vi "subFD_FLP Filtering.vi"() -> ()   [LabVIEW 2023]
uses:
  <vilib>/addons/Digital Filter Design/_Objects.llb/DFD Filter Obj.ctl
  <vilib>/addons/Digital Filter Design/_Objects.llb/DFD Filter Coef.ctl
  <vilib>/addons/Digital Filter Design/_Objects.llb/DFD Filter Structure Type Selector.ctl
  <vilib>/addons/Digital Filter Design/_Objects.llb/dfd_Internal Quantization Settings.ctl
  <vilib>/addons/Digital Filter Design/_Objects.llb/dfd_Internal Quantization Srcs.ctl
  <vilib>/addons/Digital Filter Design/_Objects.llb/DFD Coef Norm Type.ctl
  <vilib>/addons/Digital Filter Design/Process.llb/DFD Filtering (Array).vi
  <vilib>/measure/maspectr.llb/FFT Spectrum (Mag-Phase) for 1 Chan.vi
  <vilib>/addons/Digital Filter Design/NI_DigFilterLicensed.lvlib
  <vilib>/measure/NI_MAPro.lvlib
  <vilib>/Analysis/NI_AALBase.lvlib
panel:
  in  "Option":enum32{"waveform", "spectrum"}(radio)
  out "Output Signal":cluster{"f0":dbl, "df":dbl, dbl[]}(graph)
  out "Input Signal":cluster{"f0":dbl, "df":dbl, dbl[]}(graph)
  out "Successful Design?":bool
  out "filter out":T1={"mSRate_Fs"=1.0, "mSRate_Version"="1.0", "mSRate_Comments"="", "mSRate_OrgCoef"={"type"=enum."Undefined", "gain"=1.0, "coef a (k)"=[], "coef b (v)"=[]}, "mSRate_CurCoef"={"type"=enum."Undefined", "gain"=1.0, "coef a (k)"=[], "coef b (v)"=[]}, "mSRate_Quantized?"=FALSE, "mSRate_QCoef"={"type"=enum."Undefined", "gain"=1.0, "coef a (k)"=[], "coef b (v)"=[]}, "mSRate_QSettings"=[], "mSRate_Order"=0, "mSRate_Scaling"={"mSRate_ScaleByPowerOf2?"=FALSE, "mSRate_ScaleType"=enum."No Norm"}} {"mSRate_QSettings"."source" items=["Coef a/k"=0, "Coef b/v"=7, "Input"=1, "Output"=2, "Multiplicand"=3, "Product"=4, "Sum"=5, "Delay"=6, "Gain"=8]}
  in  "filter in":T1={"mSRate_Fs"=1.0, "mSRate_Version"="1.0", "mSRate_Comments"="", "mSRate_OrgCoef"={"type"=enum."Undefined", "gain"=1.0, "coef a (k)"=[], "coef b (v)"=[]}, "mSRate_CurCoef"={"type"=enum."Undefined", "gain"=1.0, "coef a (k)"=[], "coef b (v)"=[]}, "mSRate_Quantized?"=FALSE, "mSRate_QCoef"={"type"=enum."Undefined", "gain"=1.0, "coef a (k)"=[], "coef b (v)"=[]}, "mSRate_QSettings"=[], "mSRate_Order"=0, "mSRate_Scaling"={"mSRate_ScaleByPowerOf2?"=FALSE, "mSRate_ScaleType"=enum."No Norm"}} {"mSRate_QSettings"."source" items=["Coef a/k"=0, "Coef b/v"=7, "Input"=1, "Output"=2, "Multiplicand"=3, "Product"=4, "Sum"=5, "Delay"=6, "Gain"=8]}
  out "OK":bool
  in  "stop":bool
  # "Input Signal"
  # "Demo Program"
  # "Output Signal"
  # "Options"
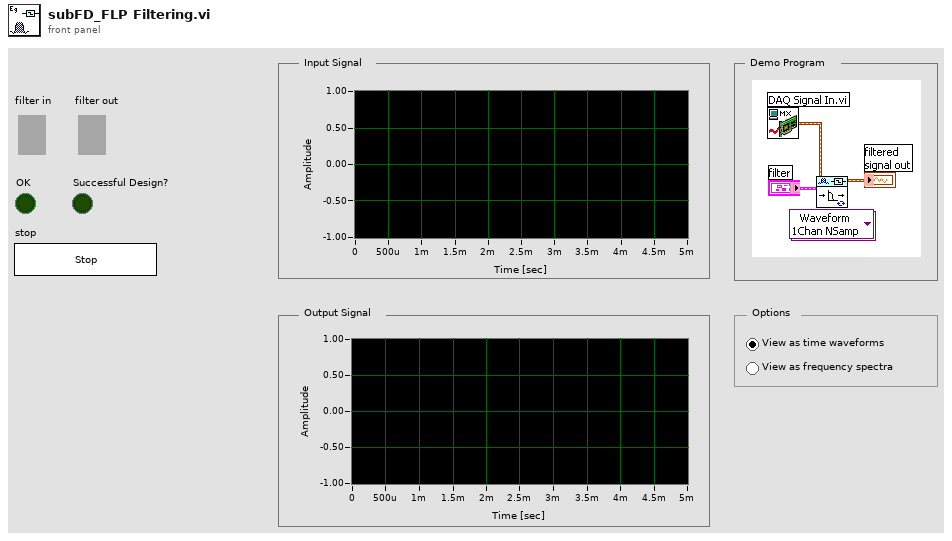
[diagram p1: front panel]
types:
  T1 = typedef "NI_DigFilterLicensed.lvlib/DFD Filter Obj.ctl" = cluster{"mSRate_Fs":dbl, "mSRate_Version":string, "mSRate_Comments":string, "mSRate_OrgCoef":T2, "mSRate_CurCoef":T2, "mSRate_Quantized?":bool, "mSRate_QCoef":T2, "mSRate_QSettings":T4[], "mSRate_Order":i32, "mSRate_Scaling":cluster{"mSRate_ScaleByPowerOf2?":bool, "mSRate_ScaleType":T6}}
  T2 = typedef "NI_DigFilterLicensed.lvlib/DFD Filter Coef.ctl" = cluster{"type":T3, "gain":dbl, "coef a (k)":dbl[], "coef b (v)":dbl[]}
  T3 = typedef "NI_DigFilterLicensed.lvlib/DFD Filter Structure Type Selector.ctl" = enum16{"Undefined", "FIR Direct Form", "FIR Direct Form Transposed", "FIR Symmetric", "FIR Antisymmetric", "IIR Direct Form I", "IIR Direct Form I Transposed", "IIR Direct Form II", "IIR Direct Form II Transposed", "IIR Cascaded Second Order Sections Form I", "IIR Cascaded Second Order Sections Form I Transposed", "IIR Cascaded Second Order Sections Form II", "IIR Cascaded Second Order Sections Form II Transposed", "Lattice Allpass (basic sections)", "Lattice Allpass (one multiplier sections)", "Lattice Allpass (normalized sections)", "Lattice AR (basic sections)", "Lattice AR (one multiplier sections)", "Lattice AR (normalized sections)", "Lattice MA (minimum phase)", "Lattice MA (maximum phase)", "Lattice ARMA (basic sections)", "Lattice ARMA (one multiplier sections)", "Lattice ARMA (normalized sections)"}
  T4 = typedef "NI_DigFilterLicensed.lvlib/dfd_Internal Quantization Settings.ctl" = cluster{"source":T5, "wl":i16, "iwl":i16, "overflow mode":enum16{"Saturation", "Wrap"}, "rounding mode":enum16{"Nearest", "Truncation"}, "signed?":bool}
  T5 = typedef "NI_DigFilterLicensed.lvlib/dfd_Internal Quantization Srcs.ctl" = u16
  T6 = typedef "NI_DigFilterLicensed.lvlib/DFD Coef Norm Type.ctl" = enum16{"No Norm", "Time Domain 1-Norm", "Time Domain 2-Norm", "Time Domain Inf-Norm"}
  T7 = cluster{"dB On (F)":bool, "unwrap phase (F)":bool, "convert to degree (F)":bool}
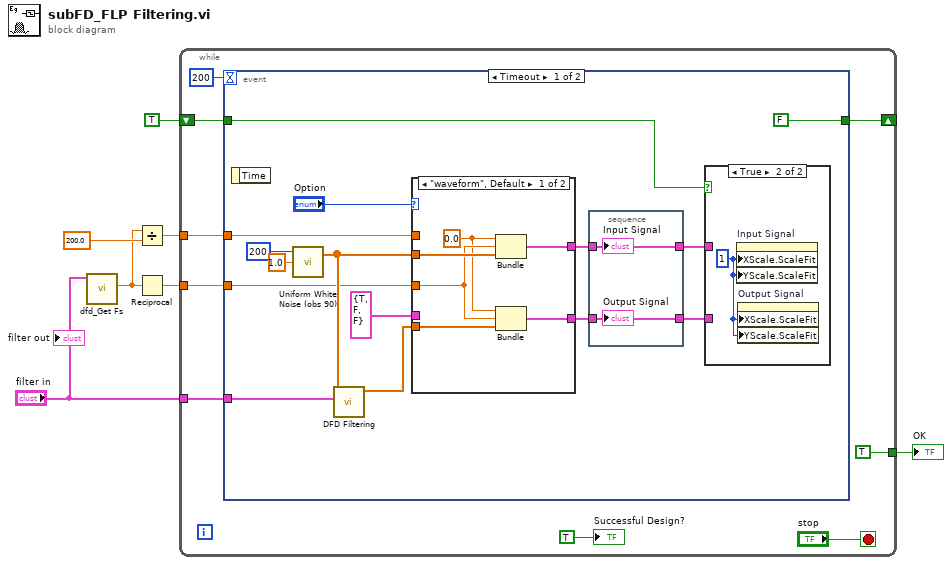
[diagram p0: block diagram]
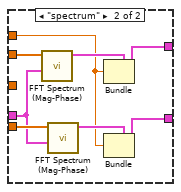
[diagram p3: hidden frame]
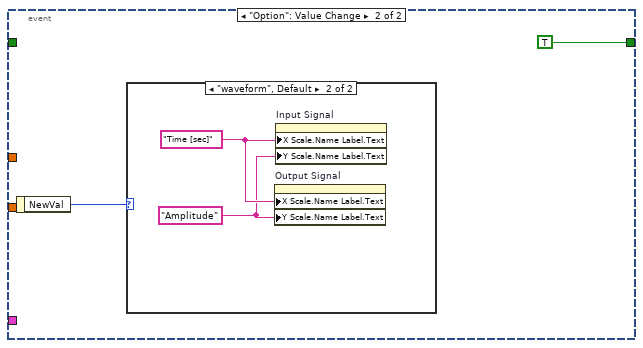
[diagram p4: hidden frame]
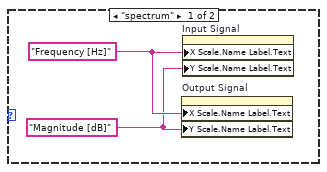
[diagram p5: hidden frame]
diagram:
  n1 = call <vilib>:"dfd_Get Fs.vi"("filter in"="filter in") -> ("fs [Hz]"=w3:dbl)  [unwired: 1 in, 9 out]
  n2 = Divide(x=w3, y=200.0) -> (x/y=w4:dbl)
  n3 = Reciprocal(x=w3) -> (1/x=w6:dbl)
  n4 = while {
    tunnel: [TRUE] -> w7
    tunnel: "filter in" -> [w12]
    tunnel: w6 -> [w11]
    tunnel: w4 -> [w10]
    shift-right: [w9] -> _
    shift-left: TRUE -> [w8]
    stop <- "stop" stop-if-true
    n5 = event shown="[0] Timeout" {
      selector: _ -> [_ _]
      dyn-events: _ -> [_ _]
      timeout: 200 -> [_ _]
      tunnel: w12 -> [w31 _]
      tunnel: w11 -> [w27 _]
      tunnel: w10 -> [w23 _]
      tunnel: [FALSE TRUE] -> w9
      tunnel: w8 -> [w19 _]
      event Timeout {
        n6 = event-data() -> ()  [unwired: 2 out]
        n7 = call <vilib>:"Uniform White Noise (obs 90).vi"("amplitude"=1.0, "samples"=200) -> ("uniform white noise"=w28:dbl[])  [unwired: 1 in, 1 out]
        n8 = call-poly <vilib>:"DFD Filtering.vi"("filter"=w31, "signal in"=w28) -> ("signal out"=w26:dbl[])  [unwired: 2 in, 7 out]
        n9 = case shown="\"waveform\", Default" "Option" {
          tunnel: w28 -> [w40 w48]
          tunnel: [w39 w42] -> w20
          tunnel: w27 -> [w38 _]
          tunnel: w26 -> [w36 w46]
          tunnel: [w35 w41] -> w21
          tunnel: w23 -> [_ w44]
          tunnel: T7 {"dB On (F)"=TRUE, "unwrap phase (F)"=FALSE, "convert to degree (F)"=FALSE} ("view") -> [_ w43]
          frame "waveform", Default {
            w37 = 0.0
            n10 = Bundle(w37, w38, "uniform white noise"=w40) -> (w39:cluster{dbl, dbl, "uniform white noise":dbl[]})  [unwired: 1 out]
            n11 = Bundle(w37, w38, "signal out"=w36) -> (w35:cluster{dbl, dbl, "signal out":dbl[]})  [unwired: 1 out]
          }
          frame "spectrum" {
            n12 = call-poly <vilib>:"FFT Spectrum (Mag-Phase).vi"("view"=w43, "time signal"=w48) -> ("magnitude"=w47:cluster{"f0":dbl, "df":dbl, "magnitude":dbl[]})  [unwired: 5 in, 4 out]
            n13 = call-poly <vilib>:"FFT Spectrum (Mag-Phase).vi"("view"=w43, "time signal"=w46) -> ("magnitude"=w45:cluster{"f0":dbl, "df":dbl, "magnitude":dbl[]})  [unwired: 5 in, 4 out]
            n14 = Bundle(cluster=w47, "df"=w44) -> (w42:cluster{"f0":dbl, "df":dbl, "magnitude":dbl[]})  [unwired: 2 out]
            n15 = Bundle(cluster=w45, "df"=w44) -> (w41:cluster{"f0":dbl, "df":dbl, "magnitude":dbl[]})  [unwired: 2 out]
          }
        }
        n16 = stacked-sequence {
          tunnel: w21 -> [w33]
          tunnel: w20 -> [w34]
          tunnel: [w34] -> w18
          tunnel: [w33] -> w17
          frame #0 {
            "Input Signal" <- w34
            "Output Signal" <- w33
          }
        }
        n17 = case shown="True" w19 {
          tunnel: w18 -> [_ _]
          tunnel: w17 -> [_ _]
          frame False {
          }
          frame True {
            w32 = u8 1 ("X Scale.Scale Fit")
            n18 = property on="Input Signal" class="WFGraph (strict)"("XScale.ScaleFit"=w32, "YScale.ScaleFit"=w32) -> ()  [unwired: 2 in, 2 out]
            n19 = property on="Output Signal" class="WFGraph (strict)"("XScale.ScaleFit"=w32, "YScale.ScaleFit"=w32) -> ()  [unwired: 2 in, 2 out]
          }
        }
      }
      event "Option": Value Change {
        n20 = event-data() -> ("NewVal"=w50:enum32{"waveform", "spectrum"})  [unwired: 1 out]
        n21 = case shown="\"waveform\", Default" w50 {
          frame "spectrum" {
            w51 = "Magnitude [dB]"
            w52 = "Frequency [Hz]"
            n22 = property on="Output Signal" class="WFGraph (strict)"("X Scale.Name Label.Text"=w52, "Y Scale.Name Label.Text"=w51) -> ()  [unwired: 2 in, 2 out]
            n23 = property on="Input Signal" class="WFGraph (strict)"("X Scale.Name Label.Text"=w52, "Y Scale.Name Label.Text"=w51) -> ()  [unwired: 2 in, 2 out]
          }
          frame "waveform", Default {
            w53 = "Amplitude"
            w54 = "Time [sec]"
            n24 = property on="Output Signal" class="WFGraph (strict)"("X Scale.Name Label.Text"=w54, "Y Scale.Name Label.Text"=w53) -> ()  [unwired: 2 in, 2 out]
            n25 = property on="Input Signal" class="WFGraph (strict)"("X Scale.Name Label.Text"=w54, "Y Scale.Name Label.Text"=w53) -> ()  [unwired: 2 in, 2 out]
          }
        }
      }
    }
    "Successful Design?" <- TRUE ("Successful Design?")
  }
  "OK" <- w7
  "filter out" <- "filter in"
